vi "Pockels-Calc sequence length in points.vi"(11 "Sequence length (ms)":dbl) -> (3 "Points length":i32)   [LabVIEW 2017]
uses:
  Global Variables/General Globals.vi
panel:
  out "In Range?":bool
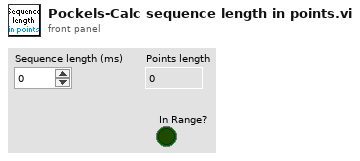
[diagram p1: front panel]
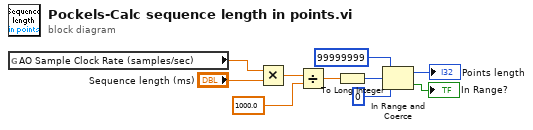
[diagram p0: block diagram]
diagram:
  n1 = global read "General Globals.vi" "AO Sample Clock Rate (samples/sec)"() -> (w1:dbl)
  n2 = Multiply(x=w1, y="Sequence length (ms)") -> (x*y=w8:dbl)
  n3 = Divide(x=w8, y=1000.0) -> (x/y=w10:dbl)
  n4 = To Long Integer(number=w10) -> (32bit integer=w6:i32)
  n5 = In Range and Coerce(upper limit=99999999, x=w6, lower limit=0) -> (coerced(x)=→"Points length":i32, In Range?=→"In Range?":bool)
